vi "RegisterMapScan.vi"(9 "Register Map":string) -> (0 "Item Array":T1[](array[typedef]), 1 "Base":u8)   [LabVIEW 2010]
doc: "This VI parses the an 8-bit register string that contains information on the register fields.\nA valid register string should contain:\n - 8 characters of 0, 1, or A-H representing the bits in the register\n - Non-programmable bits are represented with characters 0 and 1\n - Programmble bits are represented with characters A-H\n - Group settings requiring multiple-bits should use the same character.\n - Group setttings should begin with A and proceed in ascending order. Not all characters in the sequence A-H need to be used.\n - MSB bit is the left-most character in the string\n\nInputs:\nRegister Map - 8 character string representing the register settings/groupings.\n\nOutputs:\nBase - Base value of register when all programmble bits are set to 0 (A-H are replaced with 0).\nItem Array - (cluster array) contains information on each register settinging group in the register. Array[0] represents the MSB grouping.\n [cluster] - \n -> LSB (int)- LSB of the group field\n -> MSB (int)- MSB of the group field\n -> Multi? (bool) - TRUE if group field contains multiple bits"
uses:
  Controls/TYP_CtrlRegItem.ctl
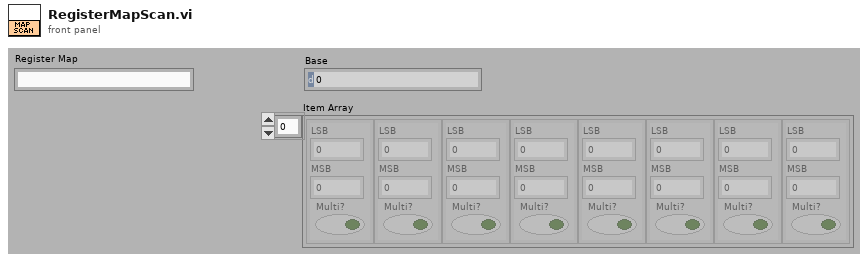
[diagram p1: front panel]
types:
  T1 = typedef "TYP_CtrlRegItem.ctl" = cluster{"LSB":u8, "MSB":u8, "Multi?":bool}
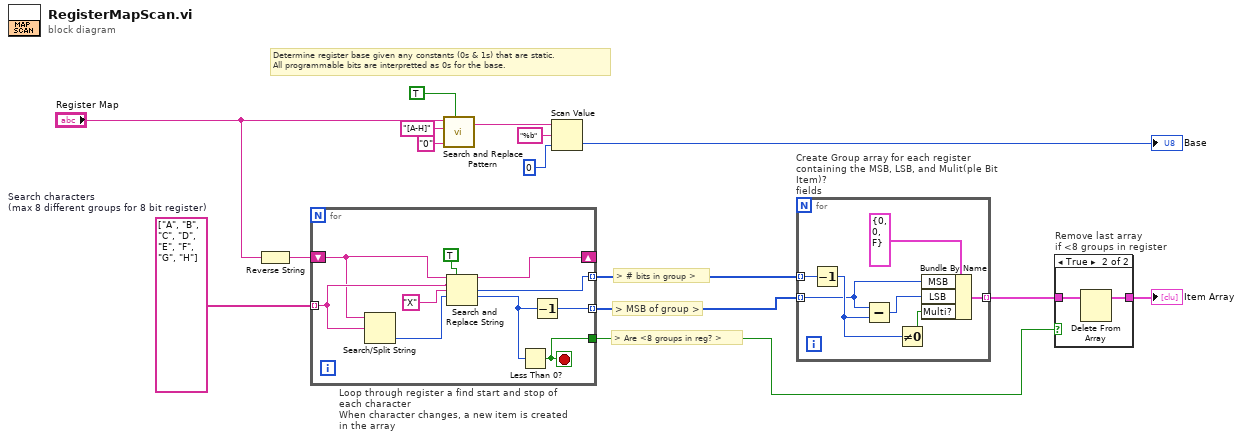
[diagram p0: block diagram]
diagram:
  w4 = string[] ["A", "B", "C", "D", "E", "F", "G", "H"]  # Search characters (max 8 different groups for 8 bit register)
  # "> Are <8 groups in reg? >"
  # "> MSB of group >"
  # "> # bits in group >"
  # "Determine register base given any constants (0s & 1s) that are static.\nAll programmable bits are interpretted as 0s for the base."
  n1 = Reverse String(1:"Register Map") -> (0:w7:string)
  n2 = for "Loop through register a find start and stop of each character\nWhen character changes, a new item is created in the array" {
    tunnel: w4 -> [w25] mode=indexing
    tunnel: [w21] -> w5 mode=indexing
    tunnel: [w19] -> w6 mode=indexing
    shift-right: [w20] -> _
    shift-left: w7 -> [w18]
    tunnel: [w16] -> w2
    stop <- w16 stop-if-true
    n3 = Search/Split String(string=w18, search string/char (-)=w25) -> (offset of match=w23:i32)  [unwired: 3 out]
    n4 = Search and Replace String(replace all?=TRUE ("replace all? (F)"), input string=w18, search string=w25, replace string="X" ("replace string (\"\")"), offset=w23) -> (result string=w20:string, number of replacements=w21:i32, offset past replacement=w17:i32)  [unwired: 1 in, 3 out]
    n5 = Less Than 0?(x=w17) -> (x < 0?=w16:bool)
    n6 = Decrement(x=w17) -> (x-1=w19:i32)
  }
  n7 = call <vilib>:"Search and Replace Pattern.vi"("string"="Register Map", "regular expression (\"\")"="[A-H]" ("regular expression (\"\")"), "replace string (\"\")"="0" ("replace string (\"\")"), "replace all? (F)"=TRUE) -> ("result string"=w10:string)  [unwired: 2 out]
  n8 = Scan Value(string=w10, format string="%b", default (0 dbl)=u8 0) -> (value=→"Base":u8)  [unwired: 1 out]
  n9 = for "Create Group array for each register\ncontaining the MSB, LSB, and Mulit(ple Bit Item)?\nfields" {
    tunnel: w6 -> [w27] mode=indexing
    tunnel: w5 -> [w31] mode=indexing
    tunnel: [w30] -> w3 mode=indexing
    n10 = Decrement(x=w31) -> (x-1=w28:i32)
    n11 = Subtract(x=w27, y=w28) -> (x-y=w26:i32)
    n12 = Not Equal To 0?(x=w28) -> (x != 0?=w29:bool)
    n13 = Bundle By Name(cluster=T1 {"LSB"=0, "MSB"=0, "Multi?"=FALSE} ("CtrlReg_Item"), "MSB"=w27, "LSB"=w26, "Multi?"=w29) -> (w30:T1)
  }
  n14 = case "Remove last array\nif <8 groups in register" shown="True" w2 {
    tunnel: [w33 w35] -> w1
    tunnel: w3 -> [w33 w34]
    frame False {
    }
    frame True {
      n15 = Delete From Array(array=w34) -> (array with subset deleted=w35:T1[])  [unwired: 2 in, 1 out]
    }
  }
  "Item Array" <- w1
